vi "Clear PCM Tasks.vi"(8 "error in (no error)":errorcluster, 11 "PCM tasks":T1) -> (0 "error out":errorcluster)   [LabVIEW 2021]
uses:
  controls/digital audio protocol/PCM tasks.ctl
  <vilib>/PDM Acquisition Toolkit/host/Classes/Tasks/PCM Output/Controls/PCM Output Task DVR.ctl
  <vilib>/PDM Acquisition Toolkit/host/Classes/Tasks/PCM Output/PCM Output Task.lvclass
  <vilib>/PDM Acquisition Toolkit/host/API/PDM Acquisition Toolkit.lvlib
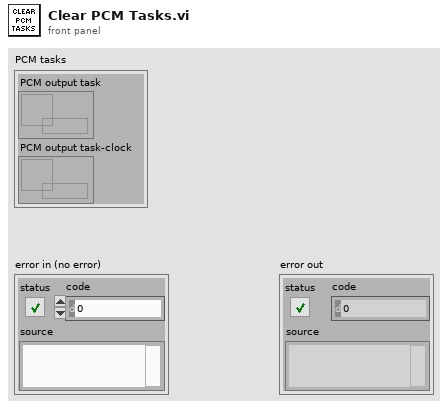
[diagram p1: front panel]
types:
  T1 = typedef "PCM tasks.ctl" = cluster{"PCM output task":T2, "PCM output task-clock":T2}
  T2 = typedef "PDM Acquisition Class Library.lvlib/PCM Output Task.lvclass/PCM Output Task DVR.ctl" = refnum<data-value>
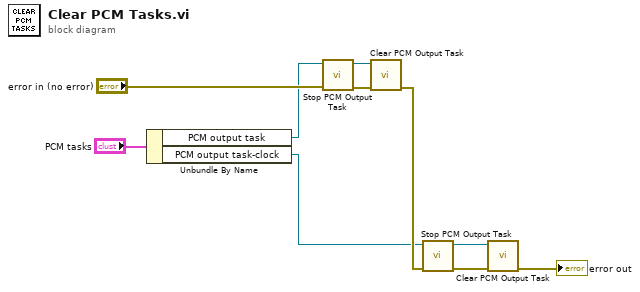
[diagram p0: block diagram]
diagram:
  n1 = Unbundle By Name("PCM tasks") -> ("PCM output task"=w2:T2, "PCM output task-clock"=w1:T2)
  n2 = call <vilib>:"Stop PCM Output Task.vi"("error in"="error in (no error)", "PCM output task In"=w2) -> ("error out"=w6:errorcluster, "PCM output task out"=w7:T2)  [unwired: 8 in]
  n3 = call <vilib>:"Clear PCM Output Task.vi"("error in"=w6, "PCM output task in"=w7) -> ("error out"=w10:errorcluster)  [unwired: 9 in]
  n4 = call <vilib>:"Stop PCM Output Task.vi"("error in"=w10, "PCM output task In"=w1) -> ("error out"=w8:errorcluster, "PCM output task out"=w9:T2)  [unwired: 8 in]
  n5 = call <vilib>:"Clear PCM Output Task.vi"("error in"=w8, "PCM output task in"=w9) -> ("error out"=→"error out":errorcluster)  [unwired: 9 in]
